vi "HEWH Start PID Conditions.vi"(8 "Error In":errorcluster, 9 "Elapsed Time (sec)":dbl) -> (0 "Error Out":errorcluster, 1 "Disable Temp Adjust?":bool)   [LabVIEW 2016]
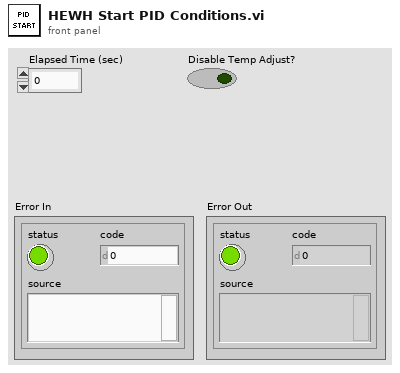
[diagram p1: front panel]
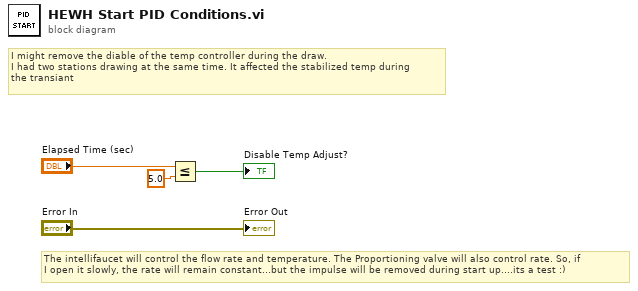
[diagram p0: block diagram]
diagram:
  # "I might remove the diable of the temp controller during the draw.\nI had two stations drawing at the same time. It affected the stabilized temp during \nthe transiant"
  # "The intellifaucet will control the flow rate and temperature. The Proportioning valve will also control rate. So, if \nI open it slowly, the rate will remain constant...but the impulse will be removed during start up....its a test :)"
  n1 = Less Or Equal?(x="Elapsed Time (sec)", y=5.0) -> (x <= y?=→"Disable Temp Adjust?":bool)
  "Error Out" <- "Error In"
